vi "总磷总氮测量流程.vi"(8 "启动参数":cluster{"总磷":bool, "总氮":bool}={"总磷"=TRUE, "总氮"=TRUE}, 9 "总氮量程模式":T1, 10 "总磷量程模式":T1, 11 "参数":T2={"站号"=1, "量程切换"=enum."AUTO", "控制命令"=enum."启动测量", "模式设置"=enum."待机", "测量间隔"=0} {"站号" items=["总磷"=1, "总氮"=2]}) -> ()   [LabVIEW 2016, in "斯坦道仪器.lvlib"]
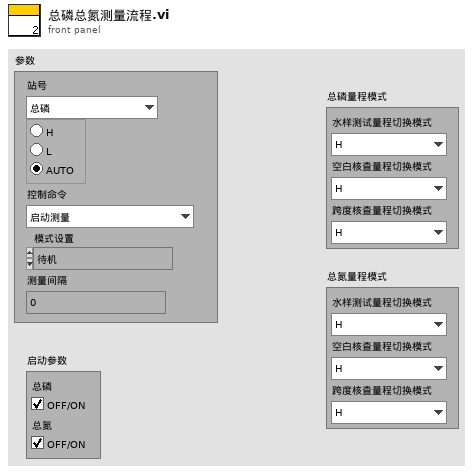
[diagram p1: front panel]
types:
  T1 = cluster{"水样测试量程切换模式":enum16{"H", "L", "AUTO"}, "空白核查量程切换模式":enum16{"H", "L", "AUTO"}, "跨度核查量程切换模式":enum16{"H", "L", "AUTO"}}
  T2 = cluster{"站号":u16, "量程切换":enum32{"H", "L", "AUTO"}, "控制命令":enum16{"启动测量", "标样核查", "零点核查", "跨度核查", "空白测试", "平行样测试", "加标回收", "空白校准", "标样校准", "初始化（清洗）", "停止测试", "仪器重启", "校时", "模式设置", "测量间隔设置"}, "模式设置":enum16{"待机", "连续模式", "周期模式", "定点模式", "受控模式", "手动模式"}, "测量间隔":u16}
  T3 = enum16{"初始化", "通电", "参数1启动", "等待参数1测试完成", "参数1测试完成", "参数1存储数据", "参数2启动", "等待参数2测试完成", "参数2测试完成", "参数2存储数据", "断电", "结束"}
  T4 = cluster{"时间标识":timestamp, "设备":string, "日志信息":string, "流程参数":string}
  T5 = cluster{"时间标识":timestamp, "监测值":sgl, "单位":u16, "数据标识":string, "因子编码":u32, "标样参考值":sgl, "F0":sgl, "F1":sgl, "F2":sgl, "F3":sgl, "F4":sgl, "F5":sgl, "F6":sgl, "F7":sgl, "X":sgl, "温度":sgl, "湿度":sgl, "量程标识":string}
  T6 = enum16{"维护数据", "水样测试", "标样核查", "零点核查", "跨度核查", "空白测试", "平行样测试", "加标回收", "空白校准", "标样校准", "初始化（清洗）"}
  T7 = enum16{"启动测量", "标样核查", "零点核查", "跨度核查", "空白测试", "平行样测试", "加标回收", "空白校准", "标样校准", "初始化（清洗）", "停止测试", "仪器重启", "校时", "模式设置", "测量间隔设置"}
  T8 = cluster{"系统时间":timestamp, "工作状态":enum16{"空闲", "水样测试", "标样核查", "零点核查", "跨度核查", "空白测试", "平行样测试", "加标回收", "空白校准", "标样校准", "初始化（清洗）"}, "测量模式":enum16{"待机", "连续模式", "周期模式", "定点模式", "受控模式", "手动模式"}, "告警代码":enum16{"无告警", "缺试剂告警", "缺水样告警", "缺蒸馏水告警", "缺标液告警", "仪表漏液告警", "标定异常告警", "超量程告警", "加热异常", "低试剂预警", "超上限告警", "超下限告警", "仪表内部其他异常", "滴定异常告警", "电极异常告警", "量程切换告警", "参数设置告警", "PH电极电位异常", "电导率电极异常", "浊度光度异常", "溶解氧电极异常", "溶解氧光强异常", "温度异常告警", "PH异常告警", "溶解氧异常告警", "电导率异常告警", "浊度异常告警", "叶绿素异常告警", "藻密度异常告警", "蓝绿藻异常告警", "ORP异常告警", "氨氮异常告警", "清洁刷异常告警", "SD卡异常告警", "蓝牙异常告警", "Wifi异常告警", "流程异常告警"}, "故障代码":enum16{"无故障", "电机故障", "温度故障", "通讯故障", "滴定故障"}, "日志代码":u16, "软件版本":u16, "F0":sgl, "F1":sgl, "F2":sgl, "F3":sgl, "T":sgl, "H":sgl, "id":u16, "flowid":u16, "量程":u16, "总磷控温温度1":sgl, "营养盐控温温度2":sgl, "ADC":sgl}
  T9 = enum16{"空闲", "水样测试", "标样核查", "零点核查", "跨度核查", "空白测试", "平行样测试", "加标回收", "空白校准", "标样校准", "初始化（清洗）"}
  T10 = cluster{"因子编码":u32, "单位":u16, "标样参考值":sgl, "水样数据时间":timestamp, "水样实测值":sgl, "水样数据标识":string, "标样数据时间":timestamp, "标样实测值":sgl, "标样数据标识":string, "空白数据时间":timestamp, "空白实测值":sgl, "空白数据标识":string, "零点核查数据时间":timestamp, "零点核查实测值":sgl, "零点核查数据标识":string, "跨度核查数据时间":timestamp, "跨度核查实测值":sgl, "跨度核查数据标识":string, "加标回收数据时间":timestamp, "加标回收实测值":sgl, "加标回收数据标识":string, "平行样数据时间":timestamp, "平行样实测值":sgl, "平行样数据标识":string, "F0":sgl, "F1":sgl, "F2":sgl, "F3":sgl, "F4":sgl, "F5":sgl, "F6":sgl, "F7":sgl, "温度":sgl, "湿度":sgl, "X值":sgl}
  T11 = cluster{"总磷跨度值":dbl, "总磷零点标准液浓度":dbl, "总磷跨度标准液浓度":dbl, "总磷标准液标准浓度":dbl, "总氮跨度值":dbl, "总氮零点标准液浓度":dbl, "总氮跨度标准液浓度":dbl, "总氮标准液标准浓度":dbl}
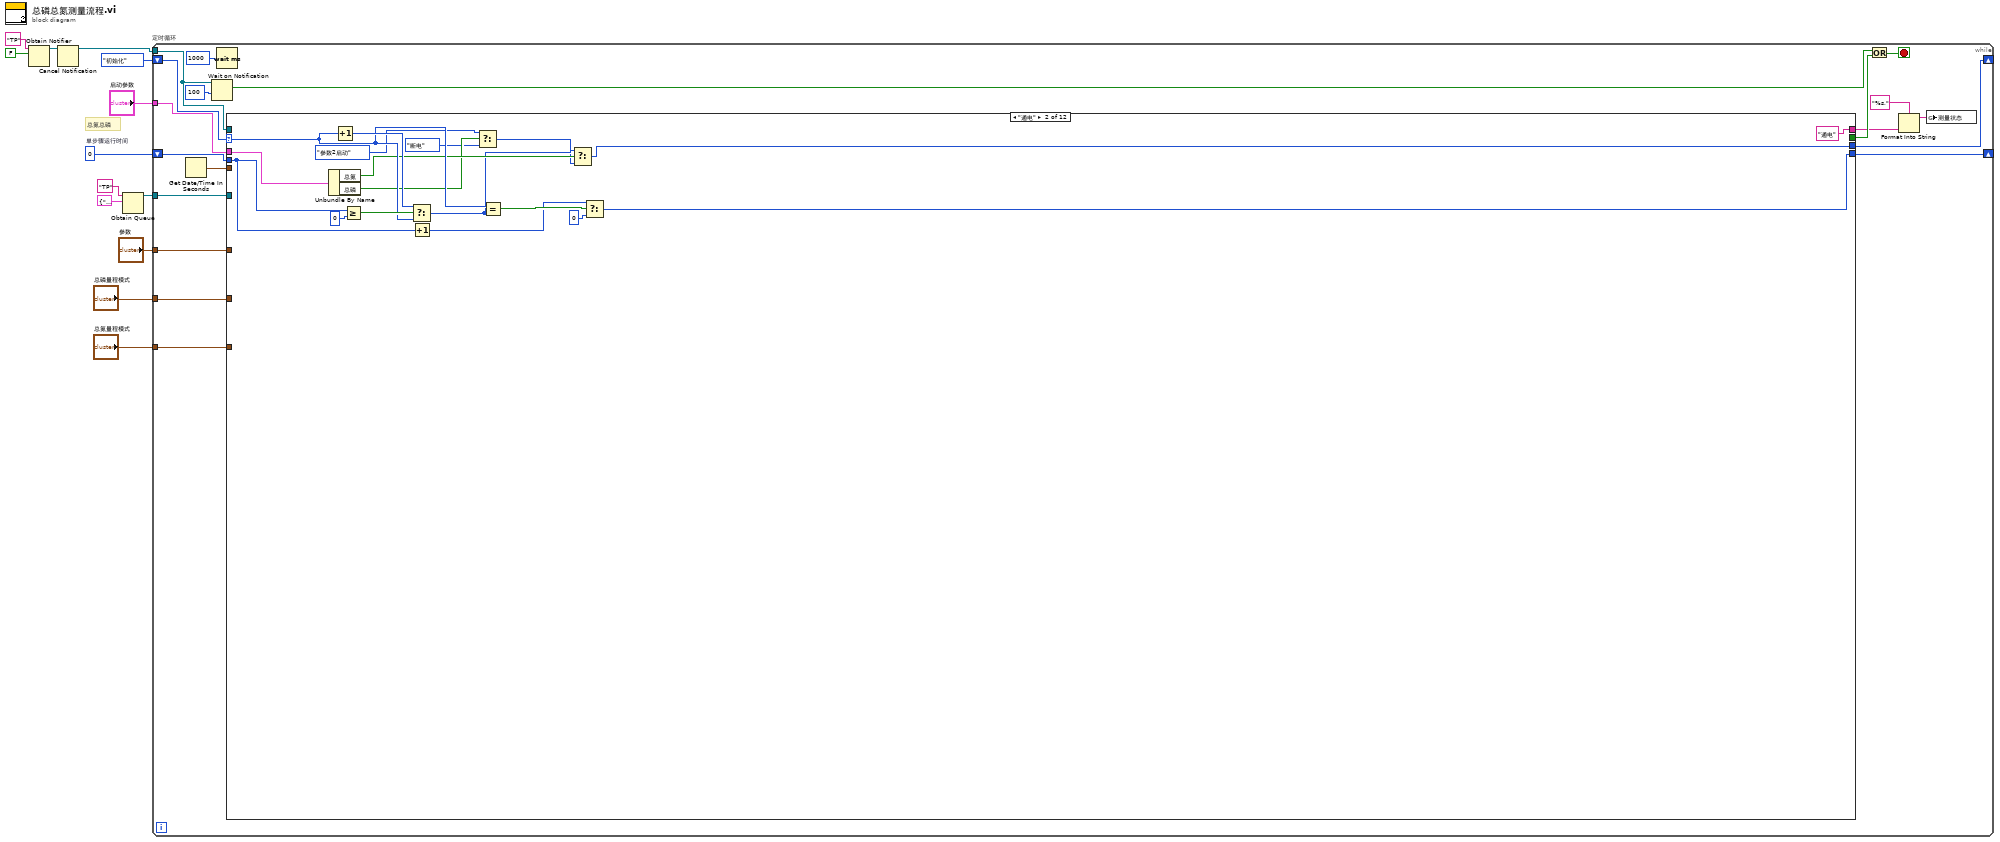
[diagram p0: block diagram]
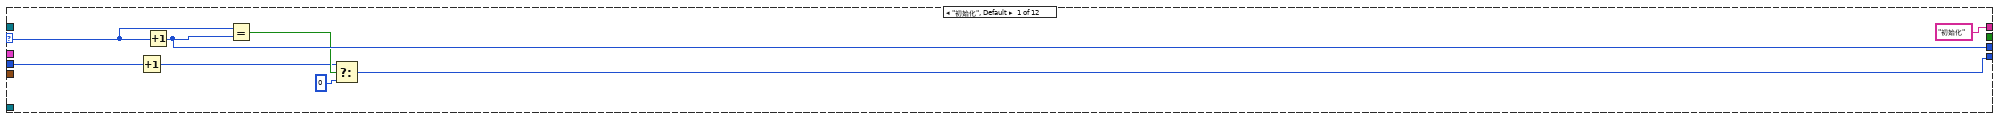
[diagram p2: hidden frame]
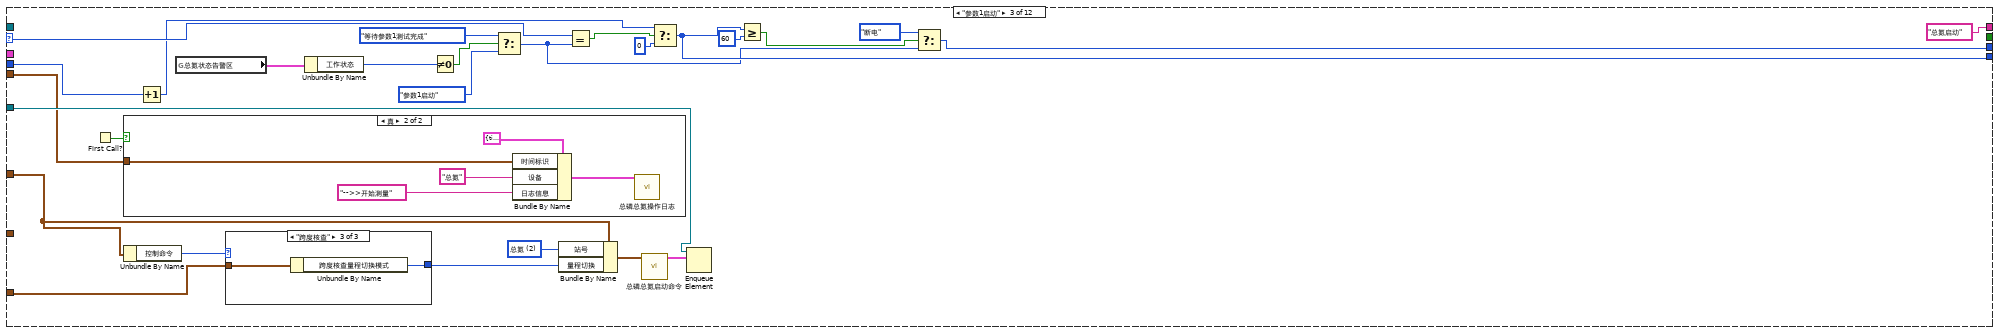
[diagram p3: hidden frame]
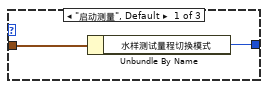
[diagram p4: hidden frame]
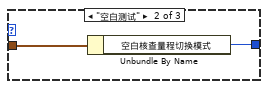
[diagram p5: hidden frame]
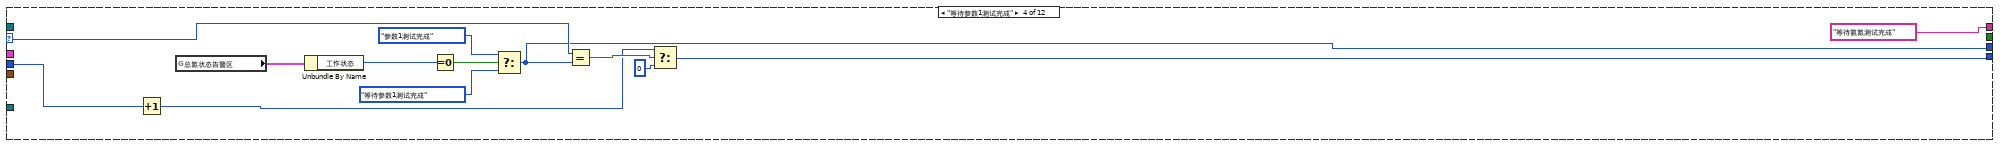
[diagram p7: hidden frame]
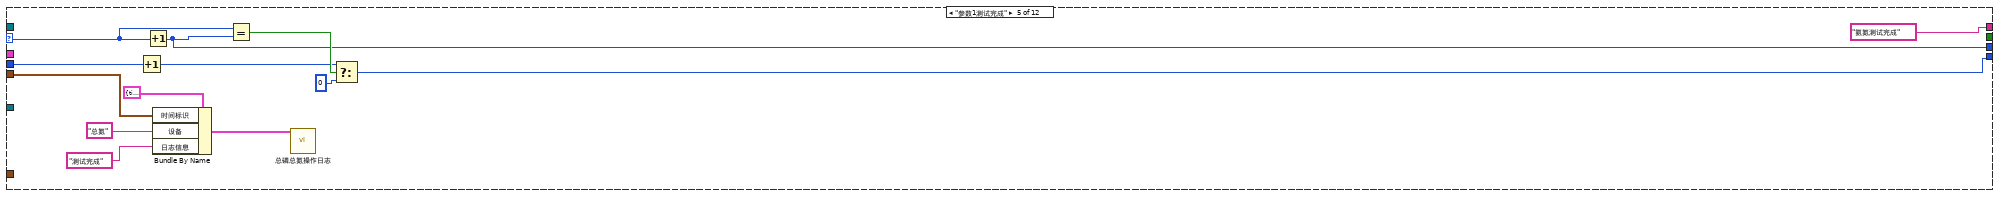
[diagram p8: hidden frame]
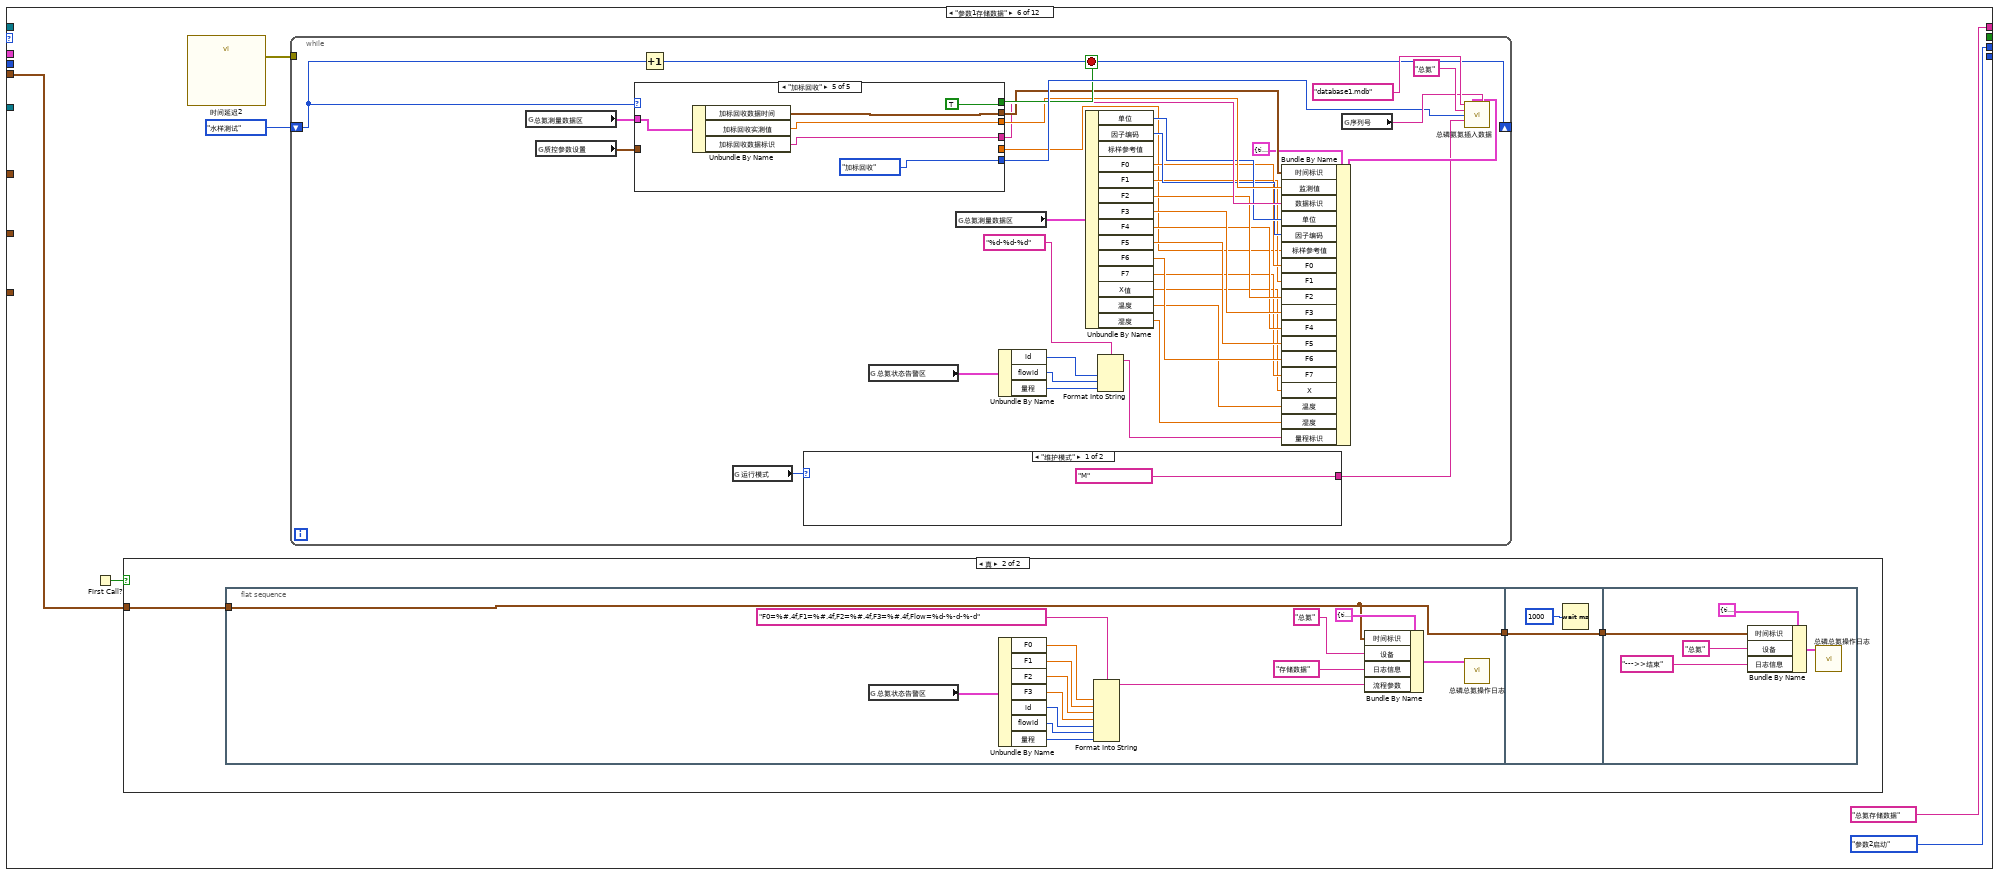
[diagram p9: hidden frame]
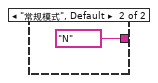
[diagram p10: hidden frame]
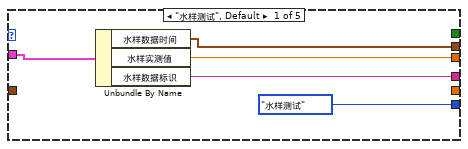
[diagram p11: hidden frame]
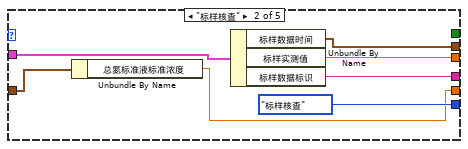
[diagram p12: hidden frame]
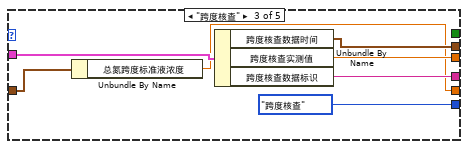
[diagram p13: hidden frame]
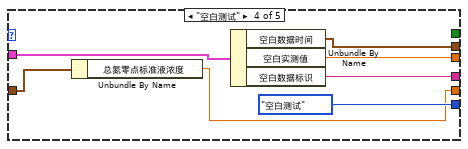
[diagram p14: hidden frame]
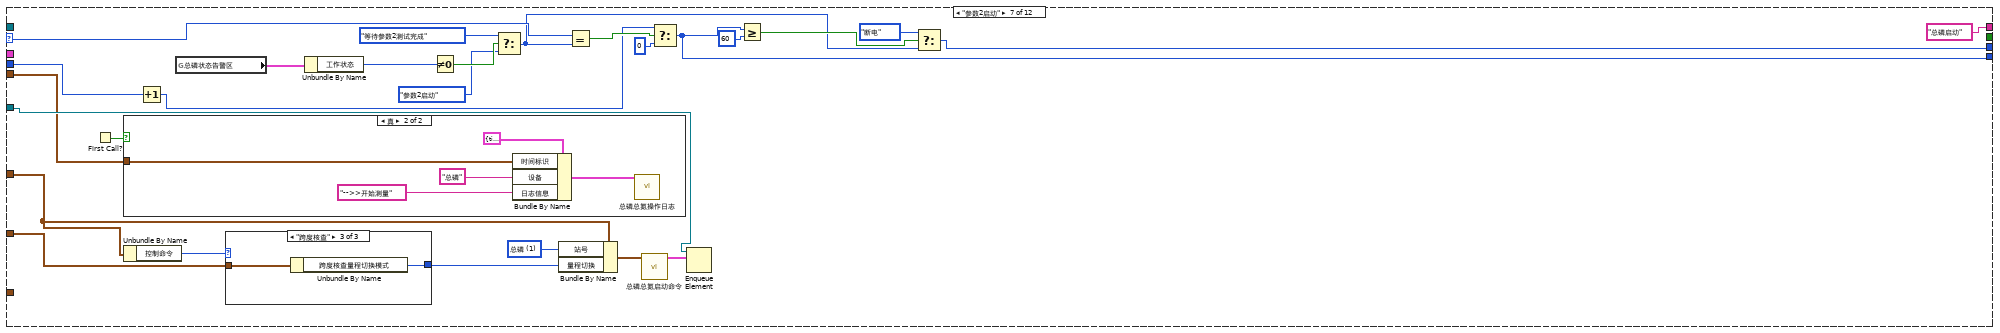
[diagram p16: hidden frame]
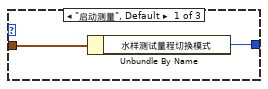
[diagram p17: hidden frame]
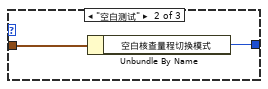
[diagram p18: hidden frame]
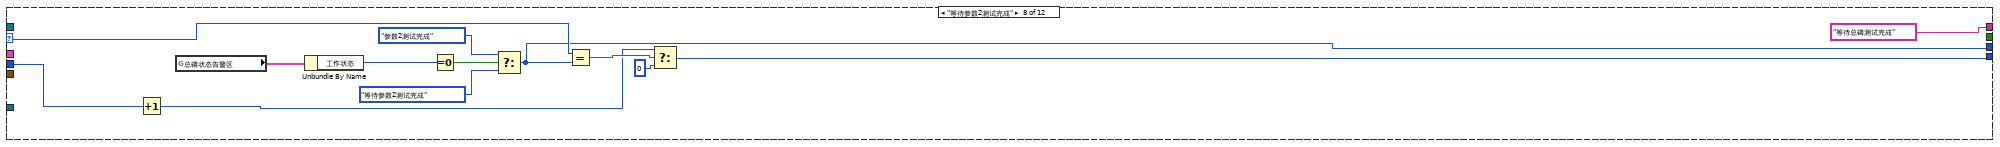
[diagram p20: hidden frame]
diagram:
  w9 = 0  # 单步骤运行时间
  # "总氮总磷"
  n1 = Obtain Notifier(name (unnamed)="TP" ("名称（未命名）"), notification data type=FALSE) -> (notifier out=w6:refnum<notifier>)  [unwired: 2 in, 2 out]
  n2 = Cancel Notification(0:w6) -> (8:w5:refnum<notifier>)  [unwired: 1 in, 2 out]
  n3 = Obtain Queue(name (unnamed)="TP" ("名称（未命名）"), element data type=cluster{"命令":string, "data":variant} {"命令"="", "data"=variant}) -> (queue out=w10:refnum<queue>)  [unwired: 3 in, 2 out]
  n4 = while "定时循环" {
    shift-right: [w31] -> _
    shift-left: T3."初始化" ("枚举") -> [w32]
    tunnel: w10 -> [w30]
    shift-right: [w28] -> _
    shift-left: w9 -> [w29]
    tunnel: w5 -> [w27]
    tunnel: "参数" -> [w22]
    tunnel: "总氮量程模式" -> [w17]
    tunnel: "总磷量程模式" -> [w15]
    tunnel: "启动参数" -> [w14]
    stop <- w23 stop-if-true
    n5 = Get Date/Time In Seconds() -> (seconds since 1Jan1904=w20:timestamp)
    n6 = Wait on Notification(notifier=w27, timeout in ms (-1)=100 ("超时毫秒(-1)")) -> (notification=w24:bool)  [unwired: 2 in, 3 out]
    n7 = Wait (ms)(milliseconds to wait=u32 1000 ("等待时间（毫秒）")) -> ()  [unwired: 1 out]
    n8 = case shown="\"通电\"" w32 {
      selector: w32 -> [w38 w52 w80 w104 w119 _ w240 w268 w284 _ w387 _]
      tunnel: [_ _ _ _ _ _ _ _ _ _ _ TRUE] -> w25
      tunnel: [w39 w45 w59 w103 w118 T3."参数2启动" ("枚举") w226 w266 w282 T3."断电" ("枚举") w386 T3."结束" ("枚举")] -> w31
      tunnel: w30 -> [_ _ w85 _ _ _ w248 _ _ _ _ w399]
      tunnel: w29 -> [w40 w53 w81 w106 w120 _ w241 w269 w285 _ w389 _]
      tunnel: [w36 w54 w64 w105 w121 _ w227 w267 w283 0 ("t") w388 0 ("t")] -> w28
      tunnel: w27 -> [_ _ _ _ _ _ _ _ _ _ _ w398]
      tunnel: w22 -> [_ _ w68 _ _ _ w234 _ _ _ _ _]
      tunnel: w20 -> [_ _ w73 _ w111 w128 w239 _ w277 w294 _ w392]
      tunnel: ["初始化" ("输入 1") "通电" ("输入 1") "总氮启动" ("输入 1") "等待氨氮测试完成" ("输入 1") "氨氮测试完成" ("输入 1") "总氮存储数据" ("输入 1") "总磷启动" ("输入 1") "等待总磷测试完成" ("输入 1") "总磷测试完成" ("输入 1") "总磷存储数据" ("输入 1") "断电" ("输入 1") "结束" ("输入 1")] -> w18
      tunnel: w17 -> [_ _ w66 _ _ _ _ _ _ _ _ _]
      tunnel: w15 -> [_ _ _ _ _ _ w225 _ _ _ _ _]
      tunnel: w14 -> [_ w48 _ _ _ _ _ _ _ _ _ _]
      frame "初始化", Default {
        n9 = Increment(x=w40) -> (x+1=w34:i32)
        n10 = Increment(x=w38) -> (x+1=w39:T3)
        n11 = Equal?(x=w38, y=w39) -> (x = y?=w37:bool)
        n12 = Select(t=w34, s=w37, f=0 ("t")) -> (s? t:f=w36:i32)
      }
      frame "通电" {
        n13 = Unbundle By Name(w48) -> ("总氮"=w47:bool, "总磷"=w44:bool)
        n14 = Increment(x=w52) -> (x+1=w56:T3)
        n15 = Greater Or Equal?(x=w53, y=0) -> (x >= y?=w57:bool)
        n16 = Select(t=w56, s=w57, f=w52) -> (s? t:f=w46:T3)
        n17 = Increment(x=w53) -> (x+1=w51:i32)
        n18 = Select(t=T3."参数2启动" ("枚举"), s=w44, f=T3."断电" ("枚举")) -> (s? t:f=w41:T3)
        n19 = Equal?(x=w52, y=w46) -> (x = y?=w55:bool)
        n20 = Select(t=w46, s=w47, f=w41) -> (s? t:f=w45:T3)
        n21 = Select(t=w51, s=w55, f=0 ("t")) -> (s? t:f=w54:i32)
      }
      frame "参数1启动" {
        w75 = u16 2 items=["总磷"=1, "总氮"=2, "氨氮"=3] ("站号")
        n22 = First Call?() -> (First Call?: T/F=w72:bool)
        n23 = case shown="真" w72 {
          tunnel: w73 -> [_ w92]
          frame False {
          }
          frame True {
            n24 = Bundle By Name(cluster=T4 {"时间标识"=timestamp(0 s since 1904-01-01), "设备"="", "日志信息"="", "流程参数"=""} ("data in"), "时间标识"=w92, "设备"="总氮", "日志信息"="-->>开始测量") -> (w96:T4)
            n25 = call "总磷总氮操作日志.vi"("data in"=w96) -> ()  [unwired: 11 in]
          }
        }
        n26 = Unbundle By Name(w68) -> ("控制命令"=w67:T7)
        n27 = Increment(x=w81) -> (x+1=w78:i32)
        n28 = global read "VAR总磷总氮全局变量.vi" "总氮状态告警区"() -> (w74:T8)
        n29 = case shown="\"跨度核查\"" w67 {
          tunnel: w66 -> [w87 w89 w91]
          tunnel: [w86 w88 w90] -> w65
          frame "启动测量", Default {
            n30 = Unbundle By Name(w87) -> ("水样测试量程切换模式"=w86:enum16{"H", "L", "AUTO"})
          }
          frame "空白测试" {
            n31 = Unbundle By Name(w89) -> ("空白核查量程切换模式"=w88:enum16{"H", "L", "AUTO"})
          }
          frame "跨度核查" {
            n32 = Unbundle By Name(w91) -> ("跨度核查量程切换模式"=w90:enum16{"H", "L", "AUTO"})
          }
        }
        n33 = Unbundle By Name(w74) -> ("工作状态"=w84:T9)
        n34 = Not Equal To 0?(x=w84) -> (x != 0?=w83:bool)
        n35 = Select(t=T3."等待参数1测试完成" ("枚举"), s=w83, f=T3."参数1启动" ("枚举")) -> (s? t:f=w61:T3)
        n36 = Bundle By Name(cluster=w68, "站号"=w75, "量程切换"=w65) -> (w76:T2)
        n37 = Equal?(x=w80, y=w61) -> (x = y?=w82:bool)
        n38 = call "总磷总氮启动命令.vi"("参数"=w76) -> ("启动命令"=w77:cluster{"命令":string, "data":variant})  [unwired: 10 in]
        n39 = Select(t=w78, s=w82, f=0 ("t")) -> (s? t:f=w64:i32)
        n40 = Enqueue Element(queue=w85, element=w77) -> ()  [unwired: 2 in, 3 out]
        n41 = Greater Or Equal?(x=w64, y=60) -> (x >= y?=w62:bool)
        n42 = Select(t=T3."断电" ("枚举"), s=w62, f=w61) -> (s? t:f=w59:T3)
      }
      frame "等待参数1测试完成" {
        n43 = Increment(x=w106) -> (x+1=w101:i32)
        n44 = global read "VAR总磷总氮全局变量.vi" "总氮状态告警区"() -> (w100:T8)
        n45 = Unbundle By Name(w100) -> ("工作状态"=w109:T9)
        n46 = Equal To 0?(x=w109) -> (x = 0?=w108:bool)
        n47 = Select(t=T3."参数1测试完成" ("枚举"), s=w108, f=T3."等待参数1测试完成" ("枚举")) -> (s? t:f=w103:T3)
        n48 = Equal?(x=w104, y=w103) -> (x = y?=w107:bool)
        n49 = Select(t=w101, s=w107, f=0 ("t")) -> (s? t:f=w105:i32)
      }
      frame "参数1测试完成" {
        n50 = Increment(x=w120) -> (x+1=w116:i32)
        n51 = Increment(x=w119) -> (x+1=w118:T3)
        n52 = Bundle By Name(cluster=T4 {"时间标识"=timestamp(0 s since 1904-01-01), "设备"="", "日志信息"="", "流程参数"=""} ("data in"), "时间标识"=w111, "设备"="总氮", "日志信息"="测试完成") -> (w115:T4)
        n53 = Equal?(x=w119, y=w118) -> (x = y?=w122:bool)
        n54 = call "总磷总氮操作日志.vi"("data in"=w115) -> ()  [unwired: 11 in]
        n55 = Select(t=w116, s=w122, f=0 ("t")) -> (s? t:f=w121:i32)
      }
      frame "参数1存储数据" {
        n56 = First Call?() -> (First Call?: T/F=w126:bool)
        n57 = case shown="真" w126 {
          tunnel: w128 -> [_ w202]
          frame False {
          }
          frame True {
            n58 = flat-sequence {
              tunnel: w202 -> [w213]
              tunnel: [w213] -> w201
              tunnel: w201 -> [w219]
              tunnel: [w219] -> w200
              tunnel: w200 -> [w220]
              frame #0 {
                n59 = global read "VAR总磷总氮全局变量.vi" "总氮状态告警区"() -> (w212:T8)
                n60 = Unbundle By Name(w212) -> ("F0"=w204:sgl, "F1"=w205:sgl, "F2"=w206:sgl, "F3"=w207:sgl, "id"=w208:u16, "flowid"=w209:u16, "量程"=w210:u16)
                n61 = Format Into String(format string="F0=%#.4f,F1=%#.4f,F2=%#.4f,F3=%#.4f,Flow=%d-%-d-%-d" ("格式字符串"), w204, w205, w206, w207, w208, w209, w210) -> (resulting string=w203:string)  [unwired: 2 in, 1 out]
                n62 = Bundle By Name(cluster=T4 {"时间标识"=timestamp(0 s since 1904-01-01), "设备"="", "日志信息"="", "流程参数"=""} ("data in"), "时间标识"=w213, "设备"="总氮", "日志信息"="存储数据", "流程参数"=w203) -> (w217:T4)
                n63 = call "总磷总氮操作日志.vi"("data in"=w217) -> ()  [unwired: 11 in]
              }
              frame #1 {
                n64 = Wait (ms)(milliseconds to wait=u32 1000 ("等待时间（毫秒）")) -> ()  [unwired: 1 out]
              }
              frame #2 {
                n65 = Bundle By Name(cluster=T4 {"时间标识"=timestamp(0 s since 1904-01-01), "设备"="", "日志信息"="", "流程参数"=""} ("data in"), "时间标识"=w220, "设备"="总氮", "日志信息"="--->>结束") -> (w221:T4)
                n66 = call "总磷总氮操作日志.vi"("data in"=w221) -> ()  [unwired: 11 in]
              }
            }
          }
        }
        n67 = call "时间延迟2"() -> ("error out"=w123:errorcluster)  [unwired: 11 in]
        n68 = while {
          shift-right: [w153] -> _
          shift-left: enum16{"水样测试", "标样核查", "跨度核查", "空白测试", "加标回收"}."水样测试" ("测量模式") -> [w154]
          tunnel: w123 -> [_]
          stop <- w155 stop-if-true
          n69 = global read "VAR总磷总氮全局变量.vi" "总氮测量数据区"() -> (w157:T10)
          n70 = global read "总磷总氮断电保存全局变量.vi" "质控参数设置"() -> (w132:T11)
          n71 = case shown="\"加标回收\"" w154 {
            tunnel: w157 -> [w168 w175 w182 w189 w194]
            tunnel: [w172 w179 w186 w193 w199] -> w151
            tunnel: [w171 w178 w185 w192 w198] -> w150
            tunnel: [w170 w177 w184 w191 w197] -> w149
            tunnel: [T6."水样测试" ("测量模式") T6."标样核查" ("测量模式") T6."跨度核查" ("测量模式") T6."空白测试" ("测量模式") T6."加标回收" ("测量模式")] -> w156
            tunnel: [_ _ _ _ TRUE] -> w155
            tunnel: w132 -> [_ w174 w181 w188 _]
            tunnel: [_ w173 w180 w187 _] -> w131
            frame "水样测试", Default {
              n72 = Unbundle By Name(w168) -> ("水样数据时间"=w172:timestamp, "水样实测值"=w171:sgl, "水样数据标识"=w170:string)
            }
            frame "标样核查" {
              n73 = Unbundle By Name(w174) -> ("总氮标准液标准浓度"=w173:dbl)
              n74 = Unbundle By Name(w175) -> ("标样数据时间"=w179:timestamp, "标样实测值"=w178:sgl, "标样数据标识"=w177:string)
            }
            frame "跨度核查" {
              n75 = Unbundle By Name(w181) -> ("总氮跨度标准液浓度"=w180:dbl)
              n76 = Unbundle By Name(w182) -> ("跨度核查数据时间"=w186:timestamp, "跨度核查实测值"=w185:sgl, "跨度核查数据标识"=w184:string)
            }
            frame "空白测试" {
              n77 = Unbundle By Name(w188) -> ("总氮零点标准液浓度"=w187:dbl)
              n78 = Unbundle By Name(w189) -> ("空白数据时间"=w193:timestamp, "空白实测值"=w192:sgl, "空白数据标识"=w191:string)
            }
            frame "加标回收" {
              n79 = Unbundle By Name(w194) -> ("加标回收数据时间"=w199:timestamp, "加标回收实测值"=w198:sgl, "加标回收数据标识"=w197:string)
            }
          }
          n80 = Increment(x=w154) -> (x+1=w153:enum16{"水样测试", "标样核查", "跨度核查", "空白测试", "加标回收"})
          n81 = global read "系统设置全局变量.vi" "运行模式"() -> (w130:enum16{"维护模式", "常规模式", "应急模式", "质控模式"})
          n82 = case shown="\"维护模式\"" w130 {
            tunnel: ["M" ("数据标记表") "N" ("数据标记表")] -> w129
            frame "维护模式" {
            }
            frame "常规模式", Default {
            }
          }
          n83 = global read "VAR总磷总氮全局变量.vi" "总氮状态告警区"() -> (w165:T8)
          n84 = global read "VAR总磷总氮全局变量.vi" "总氮测量数据区"() -> (w152:T10)
          n85 = Unbundle By Name(w165) -> ("id"=w161:u16, "flowid"=w160:u16, "量程"=w159:u16)
          n86 = Unbundle By Name(w152) -> ("单位"=w148:u16, "因子编码"=w147:u32, "F0"=w143:sgl, "F1"=w142:sgl, "F2"=w141:sgl, "F3"=w140:sgl, "F4"=w139:sgl, "F5"=w138:sgl, "F6"=w137:sgl, "F7"=w136:sgl, "X值"=w135:sgl, "温度"=w134:sgl, "湿度"=w133:sgl)  [unwired: 1 out]
          n87 = Format Into String(format string="%d-%d-%d" ("格式字符串"), w161, w160, w159) -> (resulting string=w144:string)  [unwired: 2 in, 1 out]
          n88 = Bundle By Name(cluster=T5 {"时间标识"=timestamp(0 s since 1904-01-01), "监测值"=0.0, "单位"=0, "数据标识"="", "因子编码"=0, "标样参考值"=0.0, "F0"=0.0, "F1"=0.0, "F2"=0.0, "F3"=0.0, "F4"=0.0, "F5"=0.0, "F6"=0.0, "F7"=0.0, "X"=0.0, "温度"=0.0, "湿度"=0.0, "量程标识"=""} ("data"), "时间标识"=w151, "监测值"=w150, "数据标识"=w149, "单位"=w148, "因子编码"=w147, "标样参考值"=w131, "F0"=w143, "F1"=w142, "F2"=w141, "F3"=w140, "F4"=w139, "F5"=w138, "F6"=w137, "F7"=w136, "X"=w135, "温度"=w134, "湿度"=w133, "量程标识"=w144) -> (w145:T5)
          n89 = global read "VAR总磷总氮全局变量.vi" "序列号"() -> (w158:string)
          n90 = call "总磷氨氮插入数据.vi"("database"="database1.mdb", "data"=w145, "SN"=w158, "table"="总氮", "测量模式"=w156, "数据标记表"=w129) -> ()  [unwired: 9 in, 1 out]
        }
      }
      frame "参数2启动" {
        w249 = u16 1 items=["总氮"=2, "总磷"=1] ("站号")
        n91 = First Call?() -> (First Call?: T/F=w238:bool)
        n92 = case shown="真" w238 {
          tunnel: w239 -> [_ w261]
          frame False {
          }
          frame True {
            n93 = Bundle By Name(cluster=T4 {"时间标识"=timestamp(0 s since 1904-01-01), "设备"="", "日志信息"="", "流程参数"=""} ("data in"), "时间标识"=w261, "设备"="总磷", "日志信息"="-->>开始测量") -> (w262:T4)
            n94 = call "总磷总氮操作日志.vi"("data in"=w262) -> ()  [unwired: 11 in]
          }
        }
        n95 = Unbundle By Name(w234) -> ("控制命令"=w233:T7)
        n96 = Increment(x=w241) -> (x+1=w243:i32)
        n97 = global read "VAR总磷总氮全局变量.vi" "总磷状态告警区"() -> (w242:T8)
        n98 = case shown="\"跨度核查\"" w233 {
          tunnel: w225 -> [w253 w255 w257]
          tunnel: [w252 w254 w256] -> w232
          frame "启动测量", Default {
            n99 = Unbundle By Name(w253) -> ("水样测试量程切换模式"=w252:enum16{"H", "L", "AUTO"})
          }
          frame "空白测试" {
            n100 = Unbundle By Name(w255) -> ("空白核查量程切换模式"=w254:enum16{"H", "L", "AUTO"})
          }
          frame "跨度核查" {
            n101 = Unbundle By Name(w257) -> ("跨度核查量程切换模式"=w256:enum16{"H", "L", "AUTO"})
          }
        }
        n102 = Unbundle By Name(w242) -> ("工作状态"=w247:T9)
        n103 = Not Equal To 0?(x=w247) -> (x != 0?=w246:bool)
        n104 = Select(t=T3."等待参数2测试完成" ("枚举"), s=w246, f=T3."参数2启动" ("枚举")) -> (s? t:f=w228:T3)
        n105 = Bundle By Name(cluster=w234, "站号"=w249, "量程切换"=w232) -> (w250:T2)
        n106 = Equal?(x=w240, y=w228) -> (x = y?=w245:bool)
        n107 = call "总磷总氮启动命令.vi"("参数"=w250) -> ("启动命令"=w251:cluster{"命令":string, "data":variant})  [unwired: 10 in]
        n108 = Select(t=w243, s=w245, f=0 ("t")) -> (s? t:f=w227:i32)
        n109 = Enqueue Element(queue=w248, element=w251) -> ()  [unwired: 2 in, 3 out]
        n110 = Greater Or Equal?(x=w227, y=60) -> (x >= y?=w230:bool)
        n111 = Select(t=T3."断电" ("枚举"), s=w230, f=w228) -> (s? t:f=w226:T3)
      }
      frame "等待参数2测试完成" {
        n112 = Increment(x=w269) -> (x+1=w271:i32)
        n113 = global read "VAR总磷总氮全局变量.vi" "总磷状态告警区"() -> (w270:T8)
        n114 = Unbundle By Name(w270) -> ("工作状态"=w275:T9)
        n115 = Equal To 0?(x=w275) -> (x = 0?=w274:bool)
        n116 = Select(t=T3."参数2测试完成" ("枚举"), s=w274, f=T3."等待参数2测试完成" ("枚举")) -> (s? t:f=w266:T3)
        n117 = Equal?(x=w268, y=w266) -> (x = y?=w273:bool)
        n118 = Select(t=w271, s=w273, f=0 ("t")) -> (s? t:f=w267:i32)
      }
      frame "参数2测试完成" {
        n119 = Increment(x=w285) -> (x+1=w286:i32)
        n120 = Increment(x=w284) -> (x+1=w282:T3)
        n121 = Bundle By Name(cluster=T4 {"时间标识"=timestamp(0 s since 1904-01-01), "设备"="", "日志信息"="", "流程参数"=""} ("data in"), "时间标识"=w277, "设备"="总磷", "日志信息"="测试完成") -> (w281:T4)
        n122 = Equal?(x=w284, y=w282) -> (x = y?=w288:bool)
        n123 = call "总磷总氮操作日志.vi"("data in"=w281) -> ()  [unwired: 11 in]
        n124 = Select(t=w286, s=w288, f=0 ("t")) -> (s? t:f=w283:i32)
      }
      frame "参数2存储数据" {
        n125 = First Call?() -> (First Call?: T/F=w291:bool)
        n126 = case shown="真" w291 {
          tunnel: w294 -> [_ w377]
          frame False {
          }
          frame True {
            n127 = global read "VAR总磷总氮全局变量.vi" "总磷状态告警区"() -> (w376:T8)
            n128 = Unbundle By Name(w376) -> ("F0"=w368:sgl, "F1"=w369:sgl, "F2"=w370:sgl, "F3"=w371:sgl, "id"=w372:u16, "flowid"=w373:u16, "量程"=w374:u16)
            n129 = Format Into String(format string="F0=%#.4f,F1=%#.4f,F2=%#.4f,F3=%#.4f,Flow=%d-%-d-%-d" ("格式字符串"), w368, w369, w370, w371, w372, w373, w374) -> (resulting string=w367:string)  [unwired: 2 in, 1 out]
            n130 = Bundle By Name(cluster=T4 {"时间标识"=timestamp(0 s since 1904-01-01), "设备"="", "日志信息"="", "流程参数"=""} ("data in"), "时间标识"=w377, "设备"="总磷", "日志信息"="存储数据", "流程参数"=w367) -> (w381:T4)
            n131 = call "总磷总氮操作日志.vi"("data in"=w381) -> ()  [unwired: 11 in]
          }
        }
        n132 = call "时间延迟"() -> ("error out"=w289:errorcluster)  [unwired: 11 in]
        n133 = while {
          shift-right: [w316] -> _
          shift-left: enum16{"水样测试", "标样核查", "跨度核查", "空白测试", "加标回收"}."水样测试" ("测量模式") -> [w317]
          tunnel: w289 -> [_]
          stop <- w318 stop-if-true
          n134 = global read "VAR总磷总氮全局变量.vi" "总磷测量数据区"() -> (w315:T10)
          n135 = global read "总磷总氮断电保存全局变量.vi" "质控参数设置"() -> (w297:T11)
          n136 = case shown="\"跨度核查\"" w317 {
            tunnel: w315 -> [w339 w346 w353 w360 w366]
            tunnel: [w338 w345 w352 w359 w365] -> w322
            tunnel: [w337 w344 w351 w358 w364] -> w321
            tunnel: [w336 w343 w350 w357 w363] -> w320
            tunnel: [T6."水样测试" ("测量模式") T6."标样核查" ("测量模式") T6."跨度核查" ("测量模式") T6."空白测试" ("测量模式") T6."加标回收" ("测量模式")] -> w319
            tunnel: [_ _ _ _ TRUE] -> w318
            tunnel: w297 -> [_ w341 w348 w355 _]
            tunnel: [_ w340 w347 w354 _] -> w296
            frame "水样测试", Default {
              n137 = Unbundle By Name(w339) -> ("水样数据时间"=w338:timestamp, "水样实测值"=w337:sgl, "水样数据标识"=w336:string)
            }
            frame "标样核查" {
              n138 = Unbundle By Name(w341) -> ("总磷标准液标准浓度"=w340:dbl)
              n139 = Unbundle By Name(w346) -> ("标样数据时间"=w345:timestamp, "标样实测值"=w344:sgl, "标样数据标识"=w343:string)
            }
            frame "跨度核查" {
              n140 = Unbundle By Name(w348) -> ("总磷跨度标准液浓度"=w347:dbl)
              n141 = Unbundle By Name(w353) -> ("跨度核查数据时间"=w352:timestamp, "跨度核查实测值"=w351:sgl, "跨度核查数据标识"=w350:string)
            }
            frame "空白测试" {
              n142 = Unbundle By Name(w355) -> ("总磷零点标准液浓度"=w354:dbl)
              n143 = Unbundle By Name(w360) -> ("空白数据时间"=w359:timestamp, "空白实测值"=w358:sgl, "空白数据标识"=w357:string)
            }
            frame "加标回收" {
              n144 = Unbundle By Name(w366) -> ("加标回收数据时间"=w365:timestamp, "加标回收实测值"=w364:sgl, "加标回收数据标识"=w363:string)
            }
          }
          n145 = Increment(x=w317) -> (x+1=w316:enum16{"水样测试", "标样核查", "跨度核查", "空白测试", "加标回收"})
          n146 = global read "系统设置全局变量.vi" "运行模式"() -> (w299:enum16{"维护模式", "常规模式", "应急模式", "质控模式"})
          n147 = case shown="\"维护模式\"" w299 {
            tunnel: ["M" ("数据标记表") "N" ("数据标记表")] -> w298
            frame "维护模式" {
            }
            frame "常规模式", Default {
            }
          }
          n148 = global read "VAR总磷总氮全局变量.vi" "总磷状态告警区"() -> (w330:T8)
          n149 = global read "VAR总磷总氮全局变量.vi" "总磷测量数据区"() -> (w314:T10)
          n150 = Unbundle By Name(w330) -> ("id"=w326:u16, "flowid"=w325:u16, "量程"=w324:u16)
          n151 = Unbundle By Name(w314) -> ("单位"=w332:u16, "因子编码"=w331:u32, "F0"=w300:sgl, "F1"=w301:sgl, "F2"=w302:sgl, "F3"=w303:sgl, "F4"=w304:sgl, "F5"=w305:sgl, "F6"=w306:sgl, "F7"=w307:sgl, "X值"=w308:sgl, "温度"=w309:sgl, "湿度"=w310:sgl)  [unwired: 1 out]
          n152 = Format Into String(format string="%d-%d-%d" ("格式字符串"), w326, w325, w324) -> (resulting string=w311:string)  [unwired: 2 in, 1 out]
          n153 = Bundle By Name(cluster=T5 {"时间标识"=timestamp(0 s since 1904-01-01), "监测值"=0.0, "单位"=0, "数据标识"="", "因子编码"=0, "标样参考值"=0.0, "F0"=0.0, "F1"=0.0, "F2"=0.0, "F3"=0.0, "F4"=0.0, "F5"=0.0, "F6"=0.0, "F7"=0.0, "X"=0.0, "温度"=0.0, "湿度"=0.0, "量程标识"=""} ("data"), "时间标识"=w322, "监测值"=w321, "数据标识"=w320, "单位"=w332, "因子编码"=w331, "标样参考值"=w296, "F0"=w300, "F1"=w301, "F2"=w302, "F3"=w303, "F4"=w304, "F5"=w305, "F6"=w306, "F7"=w307, "X"=w308, "温度"=w309, "湿度"=w310, "量程标识"=w311) -> (w313:T5)
          n154 = global read "VAR总磷总氮全局变量.vi" "序列号"() -> (w323:string)
          n155 = call "总磷氨氮插入数据.vi"("database"="database1.mdb", "data"=w313, "SN"=w323, "table"="总磷", "测量模式"=w319, "数据标记表"=w298) -> ()  [unwired: 9 in, 1 out]
        }
      }
      frame "断电" {
        n156 = Increment(x=w389) -> (x+1=w382:i32)
        n157 = Increment(x=w387) -> (x+1=w386:T3)
        n158 = Equal?(x=w387, y=w386) -> (x = y?=w384:bool)
        n159 = Select(t=w382, s=w384, f=0 ("t")) -> (s? t:f=w388:i32)
      }
      frame "结束" {
        n160 = Release Queue(queue=w399) -> ()  [unwired: 2 in, 3 out]
        n161 = Cancel Notification(0:w398) -> (8:w397:refnum<notifier>)  [unwired: 1 in, 2 out]
        n162 = Release Notifier(notifier=w397) -> ()  [unwired: 2 in, 3 out]
        n163 = Bundle By Name(cluster=T4 {"时间标识"=timestamp(0 s since 1904-01-01), "设备"="", "日志信息"="", "流程参数"=""} ("data in"), "时间标识"=w392, "设备"="总磷", "日志信息"="--->>结束") -> (w396:T4)
        n164 = call "总磷总氮操作日志.vi"("data in"=w396) -> ()  [unwired: 11 in]
      }
    }
    n165 = Or(x=w24, y=w25) -> (x .or. y?=w23:bool)
    n166 = Format Into String(format string="%s," ("格式字符串"), w18) -> (resulting string=w16:string)  [unwired: 2 in, 1 out]
    n167 = global write "VAR总磷总氮全局变量.vi" "测量状态"(w16) -> ()
  }
